vi "test-path-planner-basic.vi"() -> ()   [LabVIEW 2019]
uses:
  <vilib>/Rock Robotics/WPI/ThirdParty/MJansen/PathPlanner/PathPlannerTrajectory.ctl
  <vilib>/Rock Robotics/WPI/ThirdParty/MJansen/PathPlanner/PathPlannerState.ctl
  <vilib>/Rock Robotics/WPI/ThirdParty/JAS_Junk/TrajLib/ROTATION2D.ctl
  <vilib>/Rock Robotics/WPI/ThirdParty/JAS_Junk/TrajLib/TRAJ_STATE.ctl
  <vilib>/Rock Robotics/WPI/ThirdParty/JAS_Junk/TrajLib/POSE2D.ctl
  <vilib>/Rock Robotics/WPI/ThirdParty/JAS_Junk/TrajLib/TRANSLATION2D.ctl
  <vilib>/Rock Robotics/WPI/ThirdParty/MJansen/PathPlanner/PathPlannerWaypoint.ctl
  <vilib>/Rock Robotics/WPI/ThirdParty/JAS_Junk/TrajLib/Util_ApproxEquals.vi
  <vilib>/Rock Robotics/WPI/ThirdParty/JAS_Junk/TrajLib/TrajectoryState_Equals.vi
  <vilib>/Rock Robotics/WPI/ThirdParty/JAS_Junk/TrajLib/Pose_Equals.vi
  <vilib>/Rock Robotics/WPI/ThirdParty/JAS_Junk/TrajLib/Translation_Equals.vi
  <vilib>/Rock Robotics/WPI/ThirdParty/JAS_Junk/TrajLib/Rotation_Equals.vi
  <vilib>/Rock Robotics/WPI/ThirdParty/JAS_Junk/TrajLib/Util_CalcDist.vi
  <vilib>/Rock Robotics/WPI/ThirdParty/MJansen/PathPlanner/PathPlanner.lvlib
  <vilib>/Rock Robotics/WPI/ThirdParty/JAS_Junk/TrajLib/Trajectory_Library.lvlib
  <vilib>/Analysis/NI_AALBase.lvlib
panel:
  in  "Tab Control":T1(tab)
  in  "jsonReadTrajFile":string="C:\\Shares\\github\\FRC_LV_TrajLib_Util_and_Samp\\FRC_Traj_Sandbox\\PathPlannerTestPath\\Javapath1.json"
  in  "Max Velocity":dbl=3.0
  in  "Max Acceleration":dbl=2.0
  in  "stop":bool
  in  "Reversed":bool
  out "PathPlannerWayPoints":T2[](array[typedef]) {"HolonomicRotation"."SIN" format="%13.4f"; "HolonomicRotation"."COS" format="%13.4f"; "HolonomicRotation"."VALUE" format="%13.4f"; "NextControl"."Y" format="%14.3f"; "NextControl"."X" format="%14.3f"; "PrevControl"."Y" format="%14.3f"; "PrevControl"."X" format="%14.3f"; "AnchorPoint"."Y" format="%14.3f"; "AnchorPoint"."X" format="%14.3f"}
  in  "Path FileName":string="C:\\Shares\\github\\FRC_LV_TrajLib_Util_and_Samp\\FRC_Traj_Sandbox\\PathPlannerTestPath\\path1.path"
  out "LabVIEW path json read error":errorcluster
  in  "LabVIEW jsonWriteFile":string="C:\\Shares\\github\\FRC_LV_TrajLib_Util_and_Samp\\FRC_Traj_Sandbox\\PathPlannerTestPath\\LabVIEWpath1.json"
  out "Java File Read Error":errorcluster
  out "LabView Write\nJSON Error":errorcluster
  out "PathPlannerTrajectory":T5 {"States"."HolonomicRotation"."SIN" format="%13.4f"; "States"."HolonomicRotation"."COS" format="%13.4f"; "States"."HolonomicRotation"."VALUE" format="%13.4f"; "States"."AngularVelocity"."SIN" format="%13.4f"; "States"."AngularVelocity"."COS" format="%13.4f"; "States"."AngularVelocity"."VALUE" format="%13.4f"; "States"."TrajectoryState"."POSE"."ROTATION"."SIN" format="%13.4f"; "States"."TrajectoryState"."POSE"."ROTATION"."COS" format="%13.4f"; "States"."TrajectoryState"."POSE"."ROTATION"."VALUE" format="%13.4f"; "States"."TrajectoryState"."POSE"."TRANSLATION"."Y" format="%14.3f"; "States"."TrajectoryState"."POSE"."TRANSLATION"."X" format="%14.3f"; "States"."AngularAcceleration"."SIN" format="%13.4f"; "States"."AngularAcceleration"."COS" format="%13.4f"; "States"."AngularAcceleration"."VALUE" format="%13.4f"}
  out "outPathPlannerStates":T6[](array[typedef]) {"HolonomicRotation"."SIN" format="%13.4f"; "HolonomicRotation"."COS" format="%13.4f"; "HolonomicRotation"."VALUE" format="%13.4f"; "AngularVelocity"."SIN" format="%13.4f"; "AngularVelocity"."COS" format="%13.4f"; "AngularVelocity"."VALUE" format="%13.4f"; "TrajectoryState"."POSE"."ROTATION"."SIN" format="%13.4f"; "TrajectoryState"."POSE"."ROTATION"."COS" format="%13.4f"; "TrajectoryState"."POSE"."ROTATION"."VALUE" format="%13.4f"; "TrajectoryState"."POSE"."TRANSLATION"."Y" format="%14.3f"; "TrajectoryState"."POSE"."TRANSLATION"."X" format="%14.3f"; "AngularAcceleration"."SIN" format="%13.4f"; "AngularAcceleration"."COS" format="%13.4f"; "AngularAcceleration"."VALUE" format="%13.4f"}
  in  "index":i32
  out "Java_TotalTime_Sec":dbl
  out "LabVIEW_TotalTime_Sec":dbl
  out "Jave and LabVIEW \nexactly equal":bool
  out "JavaStateCount":i32
  out "LabVIEWStateCount":i32
  out "States Check":bool[](array[boolean])
  out "JavaStates":T7[](array[typedef]) {"POSE"."ROTATION"."SIN" format="%13.4f"; "POSE"."ROTATION"."COS" format="%13.4f"; "POSE"."ROTATION"."VALUE" format="%13.4f"; "POSE"."TRANSLATION"."Y" format="%14.3f"; "POSE"."TRANSLATION"."X" format="%14.3f"}
  out "LabVIEWStates":T7[](array[typedef]) {"POSE"."ROTATION"."SIN" format="%13.4f"; "POSE"."ROTATION"."COS" format="%13.4f"; "POSE"."ROTATION"."VALUE" format="%13.4f"; "POSE"."TRANSLATION"."Y" format="%14.3f"; "POSE"."TRANSLATION"."X" format="%14.3f"}
  out "Differences":T7[](array[typedef]) {"POSE"."ROTATION"."SIN" format="%13.4f"; "POSE"."ROTATION"."COS" format="%13.4f"; "POSE"."ROTATION"."VALUE" format="%13.4f"; "POSE"."TRANSLATION"."Y" format="%14.3f"; "POSE"."TRANSLATION"."X" format="%14.3f"}
  out "max time diff":dbl
  out "max vel diff":dbl
  out "max accel diff":dbl
  out "max x diff":dbl
  out "max y diff":dbl
  out "max rot diff rad":dbl
  out "max curvature diff":dbl
  out "vel mean":dbl format="%0.6f"
  out "vel std dev":dbl format="%0.6f"
  out "accel mean":dbl format="%0.6f"
  out "accel std dev":dbl format="%0.6f"
  out "Java and LabVIEW \nwithin tolerance":bool
  in  "Tolerance":dbl=1e-07 format="%#_13g"
  out "XY SPLINE":cluster{dbl[], dbl[]}[](graph)
  out "XY Graph":cluster{dbl[], dbl[]}[](graph)
  out "Sample Graph":dbl[][](graph)
  out "LabVIEW Time Plot":cluster{dbl[], dbl[]}[](graph)
  out "Java Time Plot":cluster{dbl[], dbl[]}[](graph)
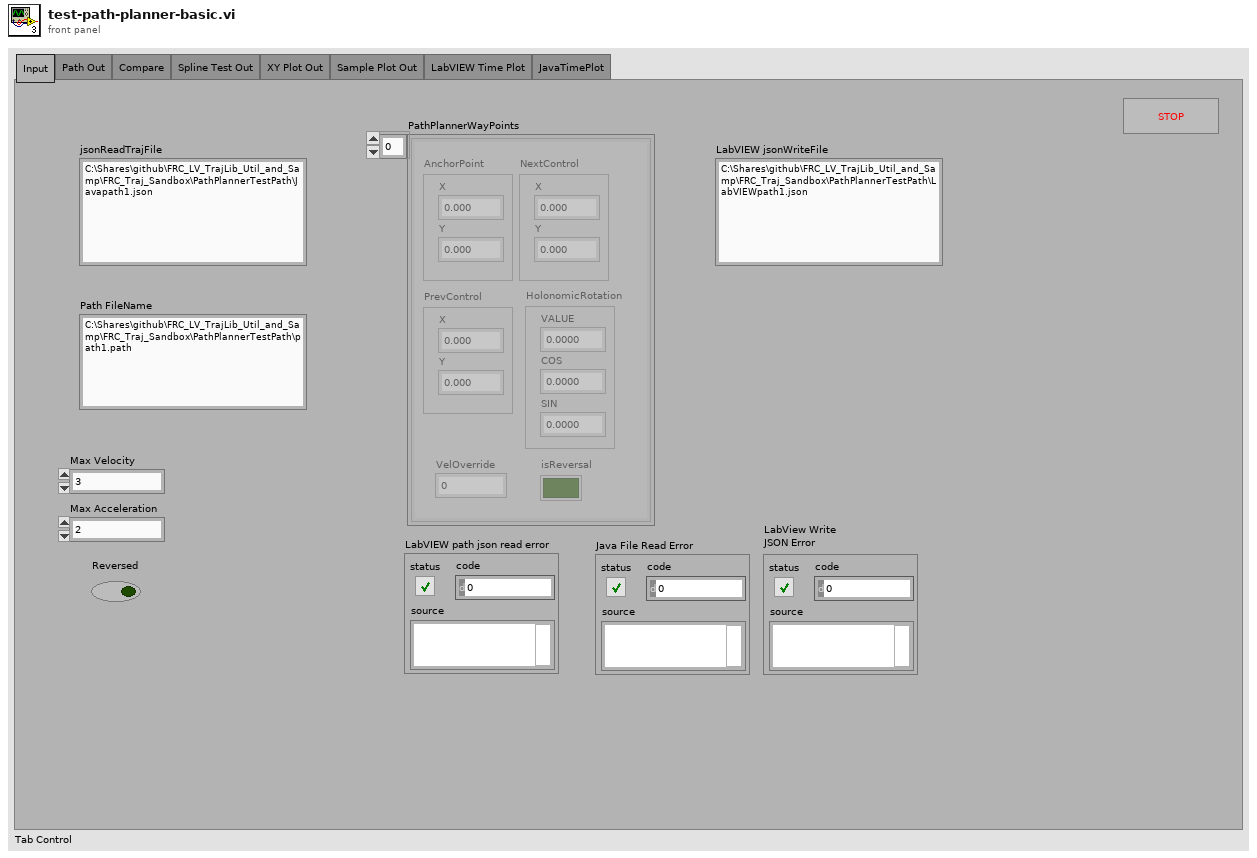
[diagram p1: front panel]
types:
  T1 = enum32{"Input", "Path Out", "Compare", "Spline Test Out", "XY Plot Out", "Sample Plot Out", "LabVIEW Time Plot", "JavaTimePlot"}
  T2 = typedef "PathPlanner.lvlib/PathPlannerWaypoint.ctl" = cluster{"AnchorPoint":T3, "PrevControl":T3, "NextControl":T3, "HolonomicRotation":T4, "VelOverride":dbl, "isReversal":bool}
  T3 = typedef "Trajectory_Library.lvlib/TRANSLATION2D.ctl" = cluster{"X":dbl, "Y":dbl}
  T4 = typedef "Trajectory_Library.lvlib/ROTATION2D.ctl" = cluster{"VALUE":dbl, "COS":dbl, "SIN":dbl}
  T5 = typedef "PathPlanner.lvlib/PathPlannerTrajectory.ctl" = cluster{"TotalTimeSeconds":dbl, "States":T6[]}
  T6 = typedef "PathPlanner.lvlib/PathPlannerState.ctl" = cluster{"AngularAcceleration":T4, "PositionMeters":dbl, "TrajectoryState":T7, "AngularVelocity":T4, "HolonomicRotation":T4, "CurveRadius":dbl, "DeltaPos":dbl}
  T7 = typedef "Trajectory_Library.lvlib/TRAJ_STATE.ctl" = cluster{"TimeSeconds":dbl, "Velocity":dbl, "Acceleration":dbl, "POSE":T8, "Curvature":dbl}
  T8 = typedef "Trajectory_Library.lvlib/POSE2D.ctl" = cluster{"TRANSLATION":T3, "ROTATION":T4}
  T9 = typedef "Trajectory_Library.lvlib/TRAJECTORY.ctl" = cluster{"TotalTImeSecs":dbl, "States":T7[]}
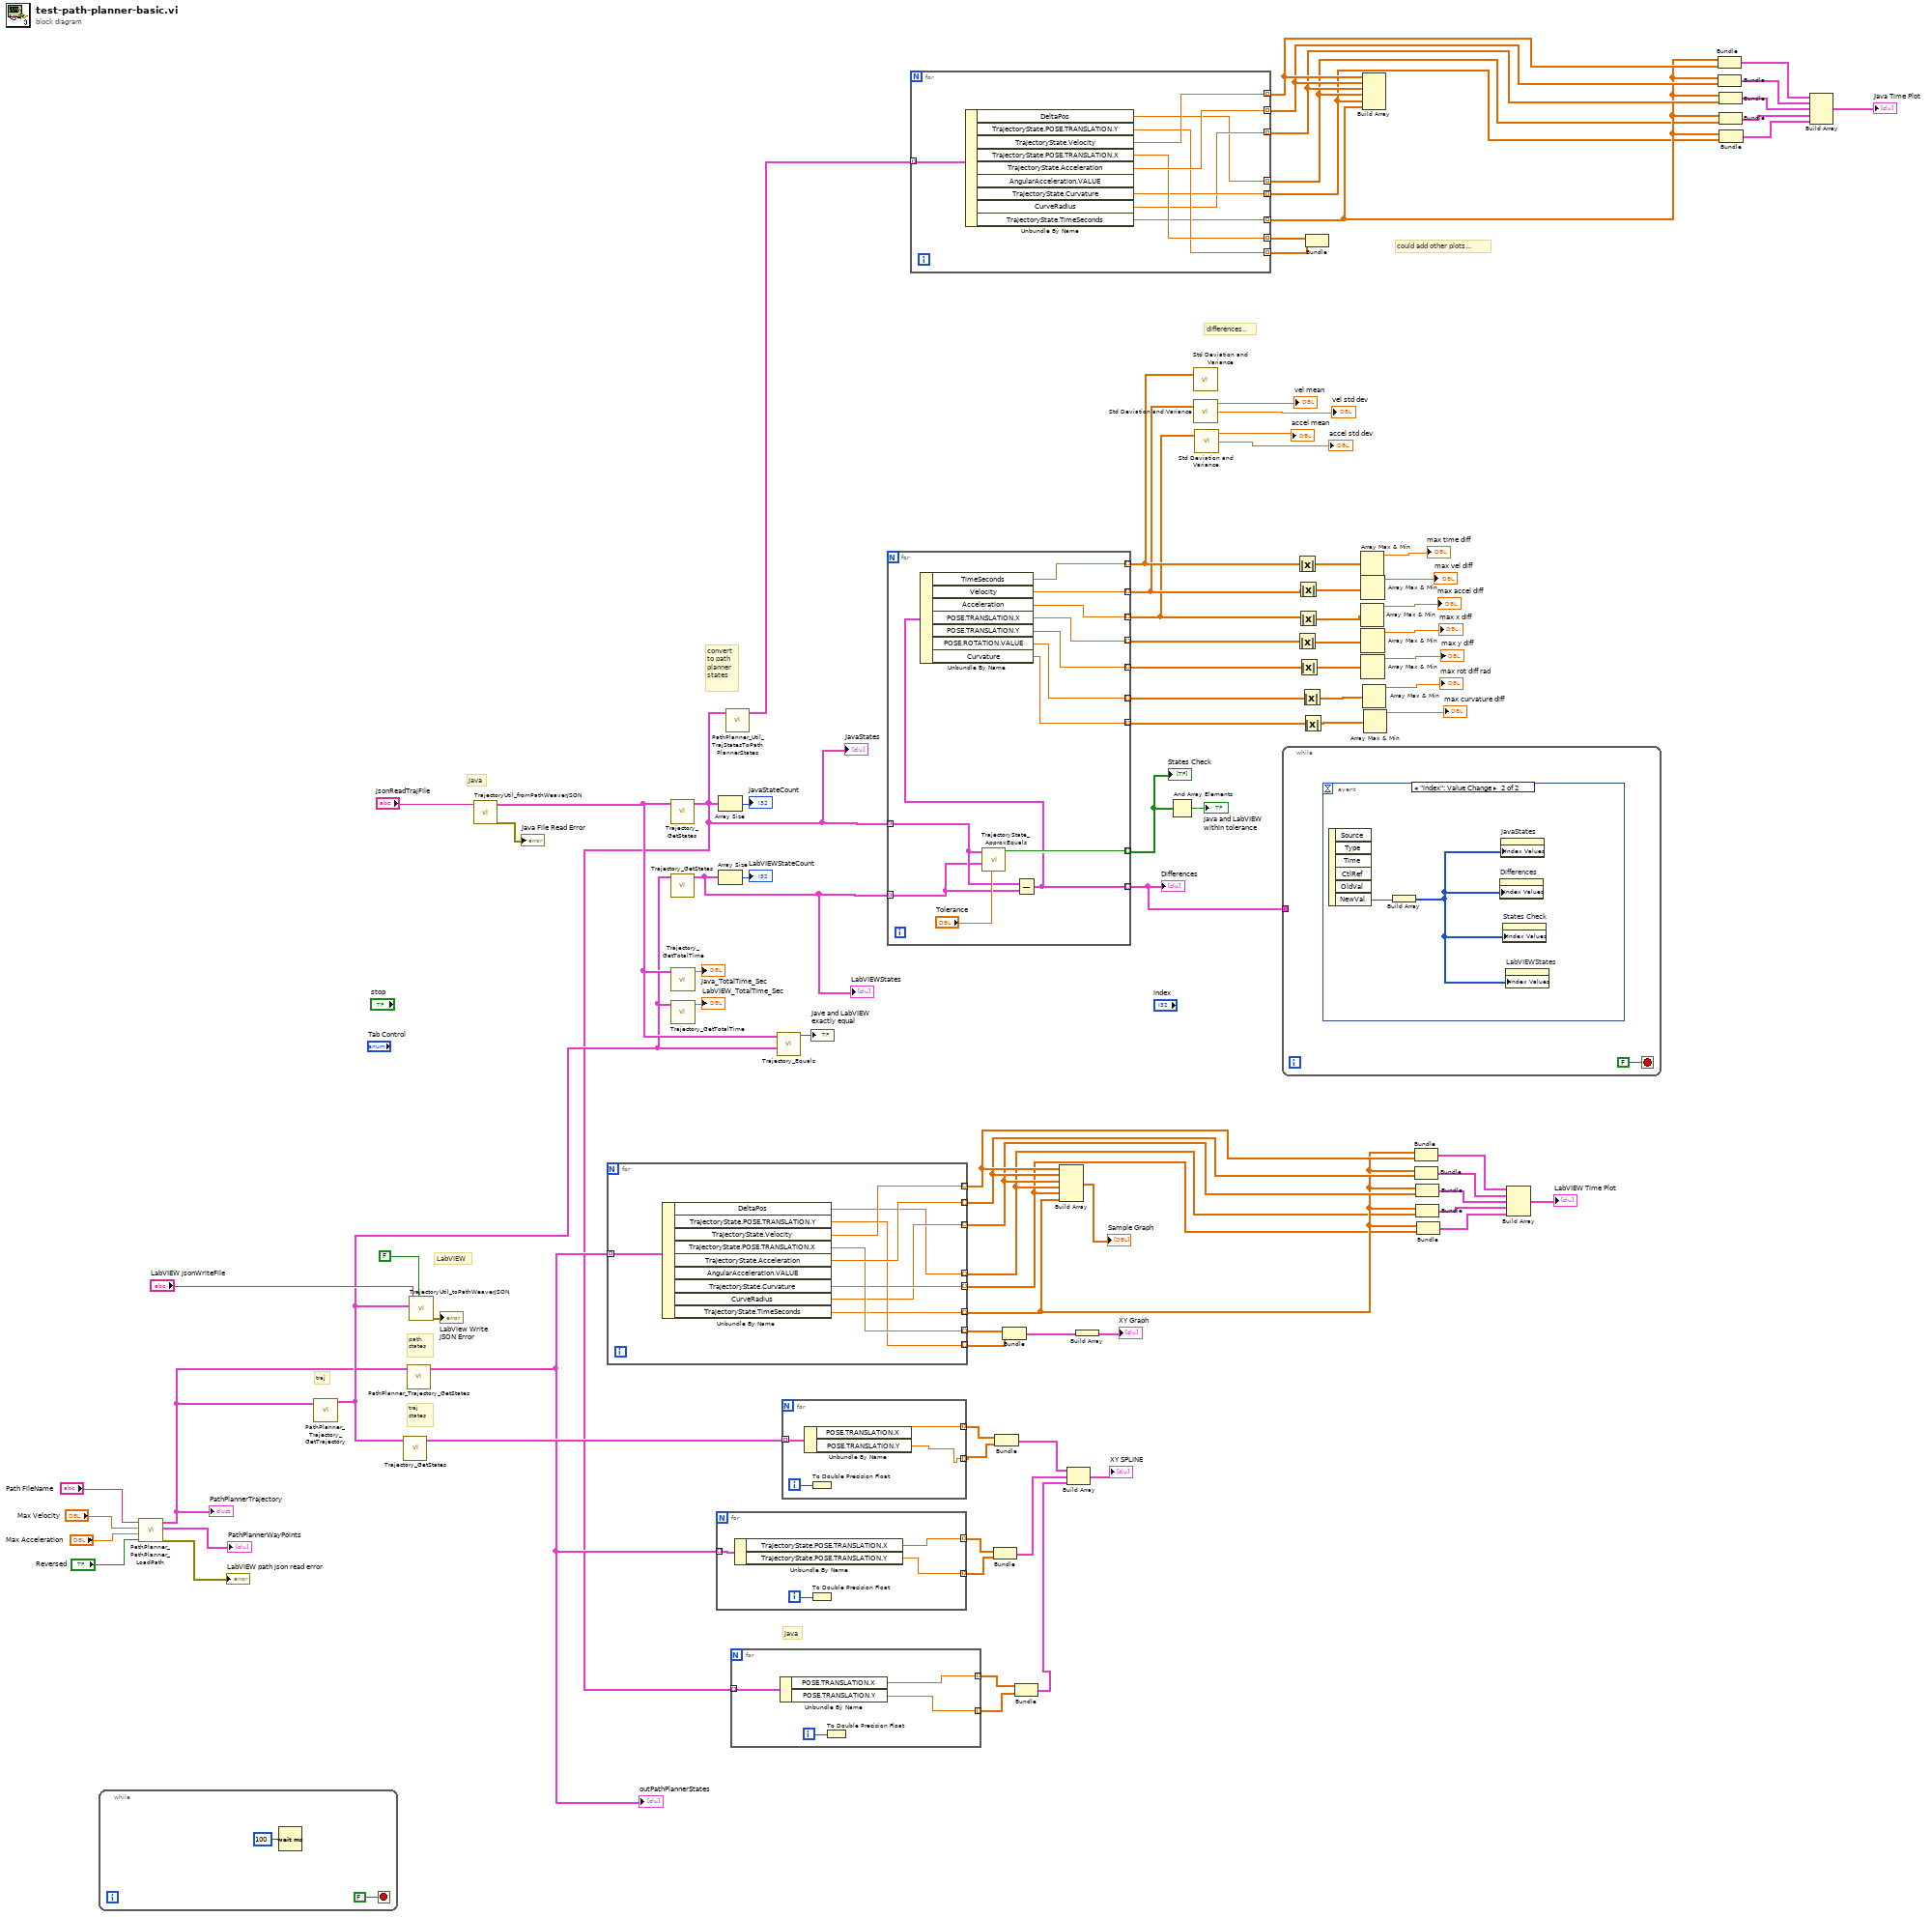
[diagram p0: block diagram]
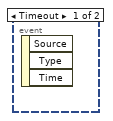
[diagram p2: hidden frame]
diagram:
  # "traj"
  # "traj\nstates"
  # "path\nstates"
  # "differences.."
  # "could add other plots..."
  # "convert\nto path\nplanner\nstates"
  # "java"
  # "LabVIEW"
  # "Java"
  n1 = while {
    stop <- FALSE stop-if-true
    n2 = Wait (ms)(milliseconds to wait=u32 100) -> ()  [unwired: 1 out]
  }
  n3 = call <vilib>:"PathPlanner_PathPlanner_LoadPath.vi"("Reversed"="Reversed", "MaxAcceleration"="Max Acceleration", "MaxVelocity"="Max Velocity", "FileName"="Path FileName") -> ("error out"=→"LabVIEW path json read error":errorcluster, "PathPlannerWayPoints"=→"PathPlannerWayPoints":T2[], "PathPlannerTrajectory"=w63:T5)  [unwired: 4 in, 1 out]
  "PathPlannerTrajectory" <- w63
  n4 = call <vilib>:"PathPlanner_Trajectory_GetTrajectory.vi"("PathPlannerTrajectory"=w63) -> ("TRAJECTORY"=w68:T9)  [unwired: 10 in]
  n5 = call <vilib>:"Trajectory_GetStates.vi"("TRAJECTORY"=w68) -> ("States"=w73:T7[])  [unwired: 10 in]
  n6 = call <vilib>:"PathPlanner_Trajectory_GetStates.vi"("PathPlannerTrajectory"=w63) -> ("PathPlannerStates"=w59:T6[])  [unwired: 10 in]
  "outPathPlannerStates" <- w59
  n7 = call <vilib>:"TrajectoryUtil_toPathWeaverJSON.vi"("AlwaysOverWrite"=FALSE, "inTRAJECTORY"=w68, "FileName"="LabVIEW jsonWriteFile") -> ("error out"=→"LabView Write\nJSON Error":errorcluster)  [unwired: 7 in, 1 out]
  n8 = call <vilib>:"TrajectoryUtil_fromPathWeaverJSON.vi"("FileName"="jsonReadTrajFile") -> ("error out"=→"Java File Read Error":errorcluster, "outTRAJECTORY"=w69:T9)  [unwired: 8 in, 1 out]
  n9 = for {
    tunnel: [w104] -> w32 mode=indexing
    tunnel: [w103] -> w31 mode=indexing
    tunnel: [w97] -> w28 mode=indexing
    tunnel: [w102] -> w92 mode=indexing
    tunnel: [w101] -> w91 mode=indexing
    tunnel: w59 -> [w100] mode=indexing
    tunnel: [w99] -> w27 mode=indexing
    tunnel: [w98] -> w30 mode=indexing
    tunnel: [w96] -> w29 mode=indexing
    n10 = Unbundle By Name(w100) -> ("DeltaPos"=w97:dbl, "TrajectoryState.POSE.TRANSLATION.Y"=w101:dbl, "TrajectoryState.Velocity"=w104:dbl, "TrajectoryState.POSE.TRANSLATION.X"=w102:dbl, "TrajectoryState.Acceleration"=w103:dbl, "TrajectoryState.Curvature"=w99:dbl, "CurveRadius"=w98:dbl, "TrajectoryState.TimeSeconds"=w96:dbl)  [unwired: 1 out]
  }
  n11 = call <vilib>:"Trajectory_GetStates.vi"("TRAJECTORY"=w69) -> ("States"=w8:T7[])  [unwired: 10 in]
  "JavaStates" <- w8
  n12 = call <vilib>:"Trajectory_GetStates.vi"("TRAJECTORY"=w68) -> ("States"=w65:T7[])  [unwired: 10 in]
  "LabVIEWStates" <- w65
  n13 = call <vilib>:"Trajectory_GetTotalTime.vi"("TRAJECTORY"=w69) -> ("TotalTime_Sec"=→"Java_TotalTime_Sec":dbl)  [unwired: 10 in]
  n14 = call <vilib>:"Trajectory_GetTotalTime.vi"("TRAJECTORY"=w68) -> ("TotalTime_Sec"=→"LabVIEW_TotalTime_Sec":dbl)  [unwired: 10 in]
  n15 = for {
    tunnel: [w107] -> w86 mode=indexing
    tunnel: w59 -> [w106] mode=indexing
    tunnel: [w105] -> w85 mode=indexing
    i -> [w108]
    n16 = Unbundle By Name(w106) -> ("TrajectoryState.POSE.TRANSLATION.X"=w107:dbl, "TrajectoryState.POSE.TRANSLATION.Y"=w105:dbl)
    n17 = To Double Precision Float(number=w108) -> ()  [unwired: 1 out]
  }
  n18 = Array Size(array=w8) -> (size(s)=→"JavaStateCount":i32)
  n19 = Array Size(array=w65) -> (size(s)=→"LabVIEWStateCount":i32)
  n20 = call "PathPlanner_Util_TrajStatesToPathPlannerStates.vi"("TrajStates"=w8) -> ("PathPlannerStates"=w7:T6[])  [unwired: 10 in]
  n21 = for {
    tunnel: [w111] -> w81 mode=indexing
    tunnel: w8 -> [w110] mode=indexing
    tunnel: [w109] -> w80 mode=indexing
    i -> [w112]
    n22 = Unbundle By Name(w110) -> ("POSE.TRANSLATION.X"=w111:dbl, "POSE.TRANSLATION.Y"=w109:dbl)
    n23 = To Double Precision Float(number=w112) -> ()  [unwired: 1 out]
  }
  n24 = call <vilib>:"Trajectory_Equals.vi"("other TRAJECTORY"=w68, "TRAJECTORY"=w69) -> ("Equals"=→"Jave and LabVIEW \nexactly equal":bool)  [unwired: 9 in]
  n25 = for {
    tunnel: [w115] -> w88 mode=indexing
    tunnel: [w114] -> w87 mode=indexing
    tunnel: w73 -> [w113] mode=indexing
    i -> [w116]
    n26 = Unbundle By Name(w113) -> ("POSE.TRANSLATION.X"=w115:dbl, "POSE.TRANSLATION.Y"=w114:dbl)
    n27 = To Double Precision Float(number=w116) -> ()  [unwired: 1 out]
  }
  n28 = for {
    tunnel: w8 -> [w126] mode=indexing
    tunnel: w65 -> [w125] mode=indexing
    tunnel: [w128] -> w6 mode=indexing
    tunnel: [w124] -> w64 mode=indexing
    tunnel: [w123] -> w40 mode=indexing
    tunnel: [w122] -> w39 mode=indexing
    tunnel: [w121] -> w38 mode=indexing
    tunnel: [w120] -> w55 mode=indexing
    tunnel: [w119] -> w56 mode=indexing
    tunnel: [w118] -> w57 mode=indexing
    tunnel: [w117] -> w58 mode=indexing
    n29 = call "TrajectoryState_ApproxEquals.vi"("Tolerance"="Tolerance", "Other TRAJ_STATE"=w125, "TRAJ_STATE"=w126) -> ("Equals"=w128:bool)  [unwired: 8 in]
    n30 = Subtract(x=w126, y=w125) -> (x-y=w124:T7)
    n31 = Unbundle By Name(w124) -> ("TimeSeconds"=w123:dbl, "Velocity"=w122:dbl, "Acceleration"=w121:dbl, "POSE.TRANSLATION.X"=w120:dbl, "POSE.TRANSLATION.Y"=w119:dbl, "POSE.ROTATION.VALUE"=w118:dbl, "Curvature"=w117:dbl)
  }
  "States Check" <- w6
  "Differences" <- w64
  n32 = for {
    tunnel: [w137] -> w19 mode=indexing
    tunnel: [w136] -> w18 mode=indexing
    tunnel: [w130] -> w15 mode=indexing
    tunnel: [w135] -> w21 mode=indexing
    tunnel: [w134] -> w20 mode=indexing
    tunnel: w7 -> [w133] mode=indexing
    tunnel: [w132] -> w14 mode=indexing
    tunnel: [w131] -> w17 mode=indexing
    tunnel: [w129] -> w16 mode=indexing
    n33 = Unbundle By Name(w133) -> ("DeltaPos"=w130:dbl, "TrajectoryState.POSE.TRANSLATION.Y"=w134:dbl, "TrajectoryState.Velocity"=w137:dbl, "TrajectoryState.POSE.TRANSLATION.X"=w135:dbl, "TrajectoryState.Acceleration"=w136:dbl, "TrajectoryState.Curvature"=w132:dbl, "CurveRadius"=w131:dbl, "TrajectoryState.TimeSeconds"=w129:dbl)  [unwired: 1 out]
  }
  n34 = Bundle(w86, w85) -> (w83:cluster{dbl[], dbl[]})  [unwired: 1 in]
  n35 = Bundle(w88, w87) -> (w84:cluster{dbl[], dbl[]})  [unwired: 1 in]
  n36 = Bundle(w92, w91) -> (w90:cluster{dbl[], dbl[]})  [unwired: 1 in]
  n37 = Bundle(w81, w80) -> (w79:cluster{dbl[], dbl[]})  [unwired: 1 in]
  n38 = Build Array(w32, w31, w30, w28, w27, w29) -> (→"Sample Graph":dbl[][])
  n39 = Build Array(w84, w83, w79) -> (→"XY SPLINE":cluster{dbl[], dbl[]}[])
  n40 = Build Array(w90) -> (→"XY Graph":cluster{dbl[], dbl[]}[])
  n41 = And Array Elements(Boolean array=w6) -> (logical AND=→"Java and LabVIEW \nwithin tolerance":bool)
  n42 = call <vilib>:"Std Deviation and Variance.vi"("X"=w40) -> ()  [unwired: 1 in, 3 out]
  n43 = call <vilib>:"Std Deviation and Variance.vi"("X"=w39) -> ("mean"=→"vel mean":dbl, "standard deviation"=→"vel std dev":dbl)  [unwired: 1 in, 1 out]
  n44 = call <vilib>:"Std Deviation and Variance.vi"("X"=w38) -> ("mean"=→"accel mean":dbl, "standard deviation"=→"accel std dev":dbl)  [unwired: 1 in, 1 out]
  n45 = while {
    tunnel: w64 -> [_]
    stop <- FALSE stop-if-true
    n46 = event shown="[1] \"index\": Value Change" {
      selector: _ -> [_ _]
      dyn-events: _ -> [_ _]
      timeout: _ -> [_ _]
      event Timeout {
        n47 = event-data() -> ()  [unwired: 1 in, 3 out]
      }
      event "index": Value Change {
        n48 = event-data() -> ("NewVal"=w140:i32)  [unwired: 1 in, 5 out]
        n49 = Build Array(w140) -> (w139:i32[])
        n50 = property on="Differences" class="Arr (strict)"("Index Values"=w139) -> ()  [unwired: 2 in, 2 out]
        n51 = property on="JavaStates" class="Arr (strict)"("Index Values"=w139) -> ()  [unwired: 2 in, 2 out]
        n52 = property on="States Check" class="Arr (strict)"("Index Values"=w139) -> ()  [unwired: 2 in, 2 out]
        n53 = property on="LabVIEWStates" class="Arr (strict)"("Index Values"=w139) -> ()  [unwired: 2 in, 2 out]
      }
    }
  }
  n54 = Absolute Value(x=w40) -> (abs(x)=w48:dbl[])
  n55 = Absolute Value(x=w55) -> (abs(x)=w51:dbl[])
  n56 = Absolute Value(x=w39) -> (abs(x)=w49:dbl[])
  n57 = Absolute Value(x=w38) -> (abs(x)=w50:dbl[])
  n58 = Absolute Value(x=w56) -> (abs(x)=w52:dbl[])
  n59 = Absolute Value(x=w57) -> (abs(x)=w53:dbl[])
  n60 = Absolute Value(x=w58) -> (abs(x)=w54:dbl[])
  n61 = Bundle(w21, w20) -> ()  [unwired: 1 in, 1 out]
  n62 = Array Max & Min(array=w48) -> (max value=→"max time diff":dbl)  [unwired: 3 out]
  n63 = Array Max & Min(array=w50) -> (max value=→"max accel diff":dbl)  [unwired: 3 out]
  n64 = Array Max & Min(array=w49) -> (max value=→"max vel diff":dbl)  [unwired: 3 out]
  n65 = Array Max & Min(array=w51) -> (max value=→"max x diff":dbl)  [unwired: 3 out]
  n66 = Array Max & Min(array=w52) -> (max value=→"max y diff":dbl)  [unwired: 3 out]
  n67 = Build Array(w19, w18, w17, w15, w14, w16) -> ()  [unwired: 1 out]
  n68 = Array Max & Min(array=w53) -> (max value=→"max rot diff rad":dbl)  [unwired: 3 out]
  n69 = Array Max & Min(array=w54) -> (max value=→"max curvature diff":dbl)  [unwired: 3 out]
  n70 = Bundle(w29, w32) -> (w26:cluster{dbl[], dbl[]})  [unwired: 1 in]
  n71 = Bundle(w29, w31) -> (w25:cluster{dbl[], dbl[]})  [unwired: 1 in]
  n72 = Bundle(w29, w30) -> (w24:cluster{dbl[], dbl[]})  [unwired: 1 in]
  n73 = Bundle(w29, w28) -> (w23:cluster{dbl[], dbl[]})  [unwired: 1 in]
  n74 = Bundle(w29, w27) -> (w22:cluster{dbl[], dbl[]})  [unwired: 1 in]
  n75 = Build Array(w26, w25, w24, w23, w22) -> (→"LabVIEW Time Plot":cluster{dbl[], dbl[]}[])
  n76 = Bundle(w16, w19) -> (w13:cluster{dbl[], dbl[]})  [unwired: 1 in]
  n77 = Bundle(w16, w18) -> (w12:cluster{dbl[], dbl[]})  [unwired: 1 in]
  n78 = Bundle(w16, w17) -> (w11:cluster{dbl[], dbl[]})  [unwired: 1 in]
  n79 = Bundle(w16, w15) -> (w10:cluster{dbl[], dbl[]})  [unwired: 1 in]
  n80 = Bundle(w16, w14) -> (w9:cluster{dbl[], dbl[]})  [unwired: 1 in]
  n81 = Build Array(w13, w12, w11, w10, w9) -> (→"Java Time Plot":cluster{dbl[], dbl[]}[])
